vi "sample block size.vi"() -> ()   [LabVIEW 2015]
panel:
  in  "Sample block size":i32=512
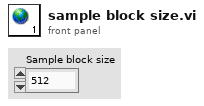
[diagram p1: front panel]
diagram:
